vi "Speed_set.vi"(1 "Speed":dbl(knob) scale=0.0..20.0, 2 "Char":i16) -> (0 "Speed":dbl)   [LabVIEW 2013]
doc: "This SubVI reads the initial speed and sets itaccording to the instruction from the keyboard and also sets a limit to the speed."
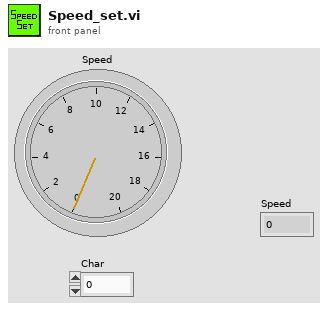
[diagram p1: front panel]
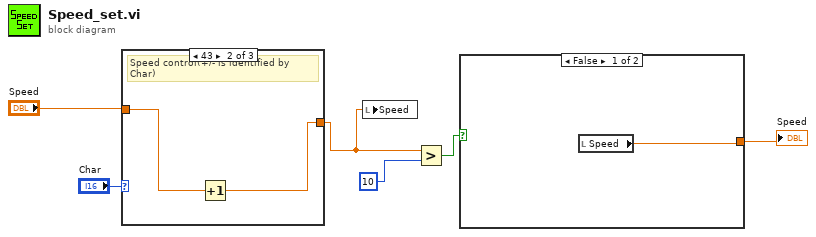
[diagram p0: block diagram]
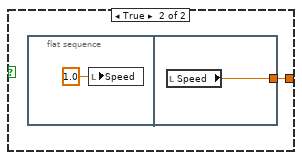
[diagram p2: hidden frame]
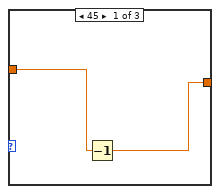
[diagram p3: hidden frame]
diagram:
  n1 = case "Case-Struktur" shown="43" "Char" {
    tunnel: [w8 w10 w11] -> w2
    tunnel: "Speed" -> [w7 w9 w11]
    frame 45 {
      n2 = Decrement(x=w7) -> (x-1=w8:dbl)
    }
    frame 43 {
      # "Speed control(+/- is identified by Char)"
      n3 = Increment(x=w9) -> (x+1=w10:dbl)
    }
    frame 55, Default {
    }
  }
  n4 = local write "Speed"(w2) -> ()
  n5 = Greater?(x=w2, y=10) -> (0:w3:bool)
  n6 = case shown="False" w3 {
    tunnel: [w12 w13] -> w1
    frame False {
      n7 = local read "Speed"() -> (w12:dbl)
    }
    frame True {
      n8 = flat-sequence {
        tunnel: [w15] -> w13
        frame #0 {
          n9 = local write "Speed"(1.0 ("Speed")) -> ()
        }
        frame #1 {
          n10 = local read "Speed"() -> (w15:dbl)
        }
      }
    }
  }
  "Speed" <- w1
